vi "SA Math - Signals Basic Statistics.vi"(0 "Signal in":waveform(dbl)[](array[waveform]), 6 "Nb Signals":i32) -> (7 "Min's":dbl[](array[numeric]), 9 "Max's":dbl[](array[numeric]), 11 "RMS":dbl[](array[numeric]), 13 "Mean / DC":dbl[](array[numeric]), 14 "Signal OUT":waveform(dbl)[](array[waveform]), 18 "Durations (msec)":dbl[](array[numeric]), 19 "Nb Samples":i32[](array[numeric]))   [LabVIEW 2022 SP3, in "GSwFormDSP.lvclass"]
uses:
  GSwFormDSP.lvclass
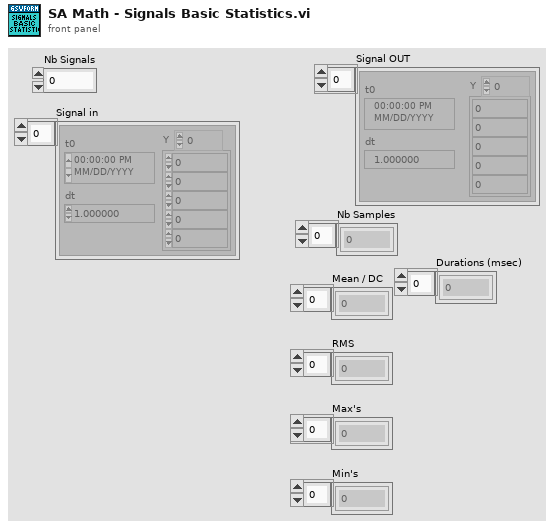
[diagram p1: front panel]
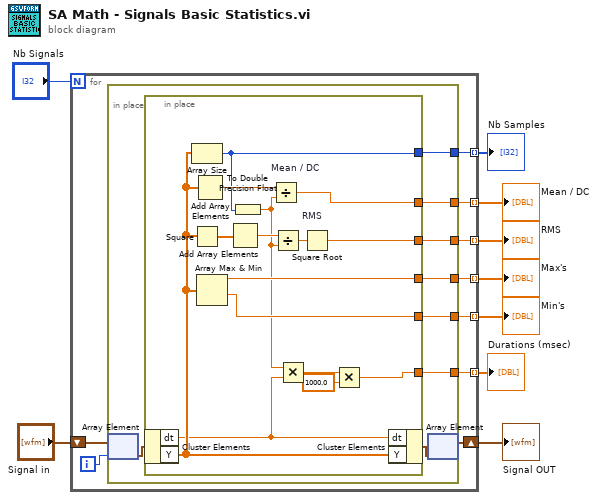
[diagram p0: block diagram]
diagram:
  n1 = for {
    N: "Nb Signals" -> [_]
    shift-right: [w16] -> w8
    shift-left: "Signal in" -> [w18]
    tunnel: [w15] -> w7 mode=indexing
    tunnel: [w14] -> w6 mode=indexing
    tunnel: [w13] -> w5 mode=indexing
    tunnel: [w12] -> w4 mode=indexing
    tunnel: [w11] -> w2 mode=indexing
    tunnel: [w10] -> w1 mode=indexing
    i -> [w17]
    n2 = in-place {
      in-place-border: [w24] -> w15
      in-place-border: [w23] -> w14
      in-place-border: [w22] -> w13
      in-place-border: [w21] -> w12
      in-place-border: [w20] -> w11
      in-place-border: [w19] -> w10
      n3 = in-place-array #1(w18, w17) -> (w26:waveform(dbl))
      n4 = in-place {
        in-place-border: [w34] -> w24
        in-place-border: [w33] -> w23
        in-place-border: [w36] -> w22
        in-place-border: [w35] -> w21
        in-place-border: [w32] -> w20
        in-place-border: [w28] -> w19
        n5 = in-place-cluster #2(w26) -> ("dt"=w30:dbl, "Y"=w37:dbl[])
        n6 = Array Size(array=w37) -> (size(s)=w32:i32)
        n7 = Square(x=w37) -> (x^2=w39:dbl[])
        n8 = Add Array Elements(numeric array=w37) -> (sum=w41:dbl)
        n9 = Array Max & Min(array=w37) -> (max value=w34:dbl, min value=w33:dbl)  [unwired: 2 out]
        n10 = Add Array Elements(numeric array=w39) -> (sum=w40:dbl)
        n11 = To Double Precision Float(number=w32) -> (double precision float=w31:dbl)
        n12 = Divide "Mean / DC"(x=w41, y=w31) -> (x/y=w35:dbl)
        n13 = Divide(x=w40, y=w31) -> (x/y=w38:dbl)
        n14 = Multiply(x=w31, y=w30) -> (x*y=w29:dbl)
        n15 = Square Root "RMS"(x=w38) -> (sqrt(x)=w36:dbl)
        n16 = Multiply(x=w29, y=1000.0) -> (x*y=w28:dbl)
        n17 = in-place-cluster #2("dt"=w30, "Y"=w37) -> (w25:waveform(dbl))
      }
      n18 = in-place-array #1(w25) -> (w16:waveform(dbl)[])  [unwired: 1 out]
    }
  }
  "Min's" <- w6
  "Max's" <- w7
  "RMS" <- w5
  "Mean / DC" <- w4
  "Signal OUT" <- w8
  "Nb Samples" <- w2
  "Durations (msec)" <- w1
